vi "Get Software Version.vi"(0 "eprom":u32, 1 "coffile":u32, 2 "vxdrev":u32, 3 "vxdver":u32, 4 "dllrev":u32, 5 "dllver":u32, 7 "error in (no error)":errorcluster) -> (20 "eprom out":u32, 21 "coffile out":u32, 22 "vxdrev out":u32, 23 "vxdver out":u32, 24 "dllrev out":u32, 25 "dllver out":u32, 26 "function return":u32, 27 "error out":errorcluster)   [LabVIEW 2014, in "atmcd32d.lvlib"]
doc: "unsigned int WINAPI GetSoftwareVersion(unsigned int * eprom, unsigned int * coffile, unsigned int * vxdrev, unsigned int * vxdver, unsigned int * dllrev, unsigned int * dllver);"
uses:
  atmcd32d.lvlib
  atmcd32d.dll
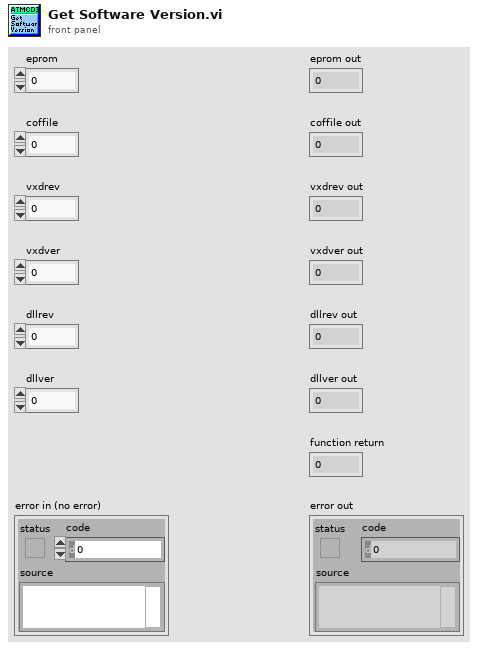
[diagram p1: front panel]
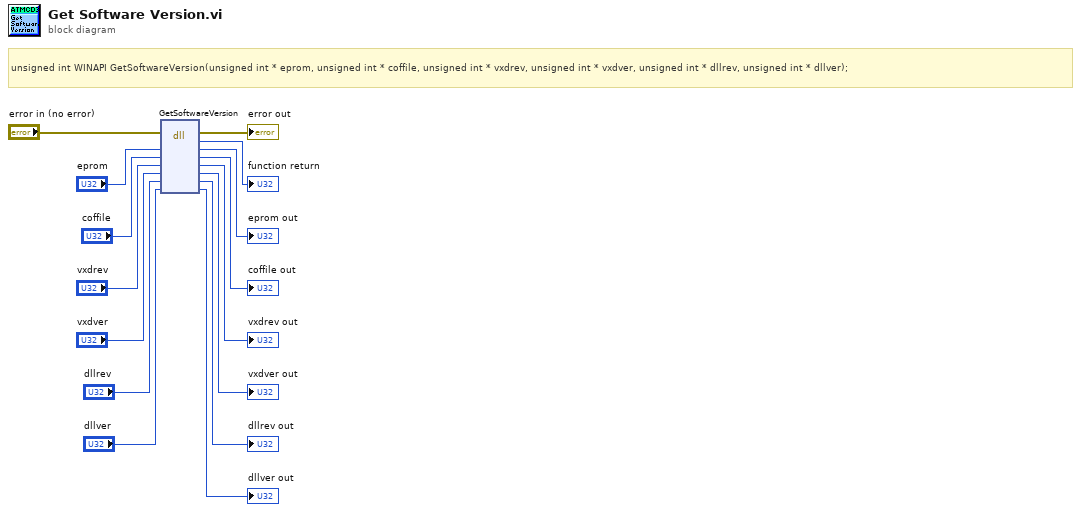
[diagram p0: block diagram]
diagram:
  # "unsigned int WINAPI GetSoftwareVersion(unsigned int * eprom, unsigned int * coffile, unsigned int * vxdrev, unsigned int * vxdver, unsigned int * dllrev, unsigned int * dllver);"
  n1 = dll-call lib="C:/Users/Bakir/Documents/Lambda2-Testing/lib/Andorlib/atmcd32d.*" fn="GetSoftwareVersion"(error in="error in (no error)", "eprom"="eprom", "coffile"="coffile", "vxdrev"="vxdrev", "vxdver"="vxdver", "dllrev"="dllrev", "dllver"="dllver") -> (error out=→"error out":errorcluster, →"function return":u32, "eprom"=→"eprom out":u32, "coffile"=→"coffile out":u32, "vxdrev"=→"vxdrev out":u32, "vxdver"=→"vxdver out":u32, "dllrev"=→"dllrev out":u32, "dllver"=→"dllver out":u32)  [unwired: 2 in, 1 out]
